vi "TANQUE_MAIN.vi"() -> ()   [LabVIEW 2017]
uses:
  <vilib>/Instr/_visa.llb/VISA Configure Serial Port (Instr).vi
  <vilib>/addons/database/Auxilliary.llb/DB Tools Format Datetime String (Time Stamp).vi
  <vilib>/addons/database/Connection.llb/DB Tools Open Connec (String).vi
  <vilib>/addons/database/NI_Database_API.lvlib
panel:
  out "SENSOR DE LLAMA":bool
  out "SENSOR DE PASO":bool
  out "hum":dbl
  out "tempp":dbl
  out "tanqueee":dbl
  in  "flow control":u16(ring) items=["None"=0, "XON/XOFF"=1, "RTS/CTS"=2, "DTR/DSR"=4]
  in  "stop bits":u16(ring)=10 items=["1.0"=10, "1.5"=15, "2.0"=20]
  in  "parity":u16(ring) items=["None", "Odd", "Even", "Mark", "Space"]
  in  "data bits":u16=8 min=5 max=8 step=1
  in  "VISA resource name":refnum<visa-resource-name>="COM1"
  in  "baud rate":u32=9600
  out "Humedity %":dbl(knob) scale=0.0..100.0
  out "Thermometer °C":dbl(slide) scale=0.0..50.0
  out "Tank":dbl(slide) scale=0.0..15.0
  out "DTH11":dbl(graph) caption="Canal Analogico 1"
  out "TERMOMETRO":dbl(graph) caption="Canal Analogico 1"
  out "ULTRASONIDO":dbl(graph) caption="Canal Analogico 1"
  # "Serial Port Config"
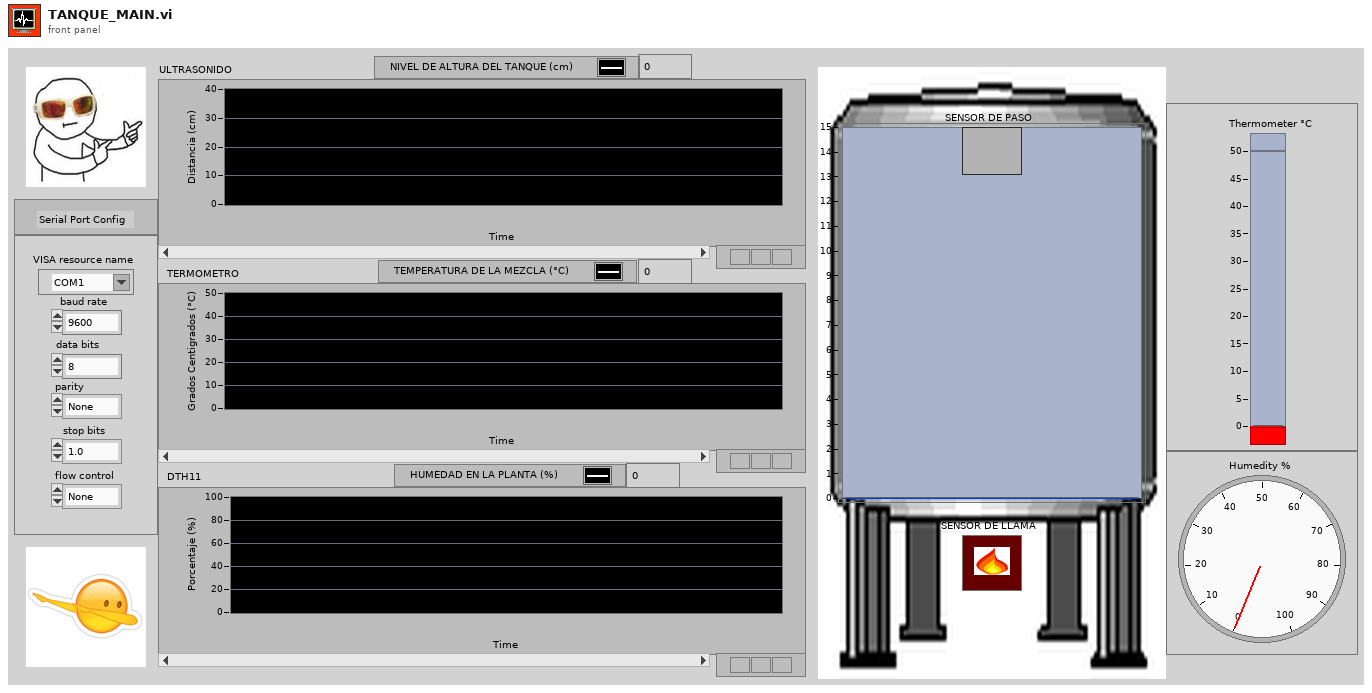
[diagram p1: front panel]
types:
  T1 = cluster{"unsigned byte array[0]":u8, "unsigned byte array[1]":u8, "unsigned byte array[2]":u8, "unsigned byte array[3]":u8, "unsigned byte array[4]":u8, "unsigned byte array[5]":u8}
  T2 = typedef "NI_Database_API.lvlib/Conn ObjectReference.ctl" = refnum<k1>
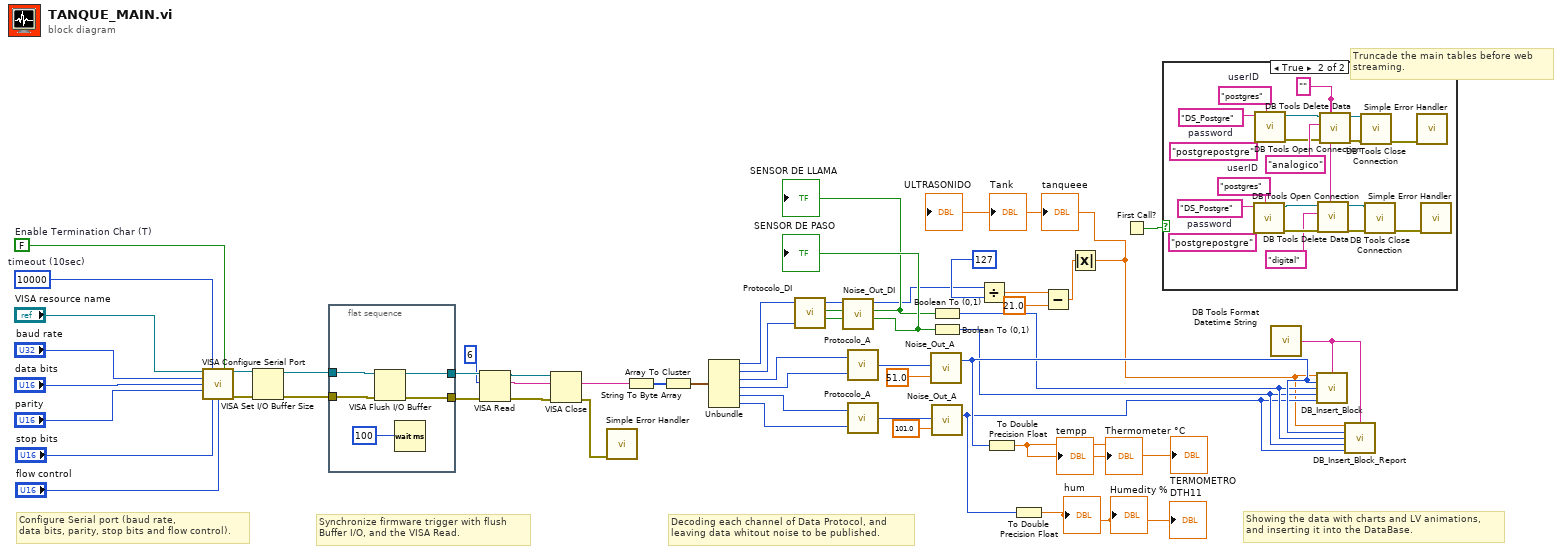
[diagram p0: block diagram]
diagram:
  w38 = FALSE  # Enable Termination Char (T)
  w39 = u32 10000  # timeout (10sec)
  # "Truncade the main tables before web \nstreaming."
  # "Showing the data with charts and LV animations,\nand inserting it into the DataBase."
  # "Decoding each channel of Data Protocol, and \nleaving data whitout noise to be published."
  # "Synchronize firmware trigger with flush \nBuffer I/O, and the VISA Read."
  # "Configure Serial port (baud rate,\ndata bits, parity, stop bits and flow control)."
  n1 = call-poly "VISA Configure Serial Port"("VISA resource name"="VISA resource name", "timeout (10sec)"=w39, "Enable Termination\nChar (T)"=w38, "baud rate (9600)"="baud rate", "data bits (8)"="data bits", "parity (0:none)"="parity", "stop bits (10: 1 bit)"="stop bits", "flow control (0:none)"="flow control") -> ("VISA resource name out"=w34:refnum<visa-resource-name>, "error out"=w33:errorcluster)  [unwired: 6 in]
  n2 = VISA Set I/O Buffer Size(VISA resource name=w34, error in (no error)=w33) -> (VISA resource name out=w32:refnum<visa-resource-name>, error out=w31:errorcluster)  [unwired: 2 in]
  n3 = flat-sequence {
    tunnel: w32 -> [w55]
    tunnel: w31 -> [w54]
    tunnel: [w53] -> w30
    tunnel: [w52] -> w29
    frame #0 {
      n4 = VISA Flush I/O Buffer(VISA resource name=w55, error in (no error)=w54) -> (VISA resource name out=w53:refnum<visa-resource-name>, error out=w52:errorcluster)  [unwired: 1 in]
      n5 = Wait (ms)(milliseconds to wait=u32 100) -> ()  [unwired: 1 out]
    }
  }
  n6 = VISA Read(VISA resource name=w30, byte count=u32 6, error in (no error)=w29) -> (VISA resource name out=w27:refnum<visa-resource-name>, read buffer=w25:string, error out=w26:errorcluster)  [unwired: 1 out]
  n7 = VISA Close(VISA resource name=w27, error in (no error)=w26) -> (error out=w28:errorcluster)
  n8 = call <vilib>:"Simple Error Handler.vi"("error in (no error)"=w28) -> ()  [unwired: 4 in, 5 out]
  n9 = String To Byte Array(string=w25) -> (unsigned byte array=w50:u8[])
  n10 = Array To Cluster(array=w50) -> (cluster=w49:T1)
  n11 = Unbundle(w49) -> ("unsigned byte array[0]"=w48:u8, "unsigned byte array[1]"=w47:u8, "unsigned byte array[2]"=w46:u8, "unsigned byte array[3]"=w45:u8, "unsigned byte array[4]"=w44:u8, "unsigned byte array[5]"=w43:u8)
  n12 = call "Protocolo_DI.vi"("Trama2"=w47, "Trama1"=w48) -> ("Digital2"=w9:bool, "Digital1"=w10:bool, "Analogico"=w11:u32)  [unwired: 1 in]
  n13 = call "Noise_Out_DI.vi"("D2"=w9, "D1"=w10, "IN"=w11) -> ("DOUT_2"=w14:bool, "DOUT_1"=w13:bool, "OUT"=w12:u32)  [unwired: 1 in, 1 out]
  "SENSOR DE PASO" <- w14
  "SENSOR DE LLAMA" <- w13
  n14 = call "Protocolo_A.vi"("Trama2"=w45, "Trama1"=w46) -> ("Analogico"=w18:u32)
  n15 = call "Protocolo_A.vi"("Trama2"=w43, "Trama1"=w44) -> ("Analogico"=w15:u32)
  n16 = call "Noise_Out_A.vi"("pico inalcanzable"=51.0, "IN"=w18) -> ("OUT"=w6:u32)  [unwired: 1 out]
  n17 = Boolean To (0,1)(Boolean=w13) -> (0, 1=w5:i16)
  n18 = Boolean To (0,1)(Boolean=w14) -> (0, 1=w4:i16)
  n19 = call "Noise_Out_A.vi"("pico inalcanzable"=101.0, "IN"=w15) -> ("OUT"=w3:u32)  [unwired: 1 out]
  n20 = Divide(x=w12, y=u32 127 ("x")) -> (x/y=w23:dbl)
  n21 = To Double Precision Float(number=w6) -> (double precision float=→"TERMOMETRO" →"Thermometer °C" →"tempp":dbl)
  n22 = To Double Precision Float(number=w3) -> (double precision float=→"DTH11" →"Humedity %" →"hum":dbl)
  n23 = Subtract(x=w23, y=21.0) -> (x-y=w2:dbl)
  n24 = Absolute Value(x=w2) -> (abs(x)=w1:dbl)
  "ULTRASONIDO" <- w1
  "Tank" <- w1
  "tanqueee" <- w1
  n25 = First Call?() -> (First Call?: T/F=w8:bool)
  n26 = case shown="True" w8 {
    frame False {
    }
    frame True {
      w56 = "" ("condition")
      (unwired) "postgrepostgre"  # password
      w70 = "postgres"  # userID
      (unwired) "postgrepostgre"  # password
      w72 = "postgres"  # userID
      n27 = call-poly <vilib>:"DB Tools Open Connection.vi"("userID"=w72, "connection information"="DS_Postgre") -> ("error out"=w65:errorcluster, "connection reference"=w64:T2)  [unwired: 6 in]
      n28 = call-poly <vilib>:"DB Tools Open Connection.vi"("userID"=w70, "connection information"="DS_Postgre") -> ("error out"=w66:errorcluster, "connection reference"=w67:T2)  [unwired: 6 in]
      n29 = call <vilib>:"DB Tools Delete Data.vi"("condition"=w56, "error in (no error)"=w65, "table"="digital", "connection reference"=w64) -> ("error out"=w59:errorcluster, "connection reference out"=w60:T2)  [unwired: 6 in]
      n30 = call <vilib>:"DB Tools Delete Data.vi"("condition"=w56, "error in (no error)"=w66, "table"="analogico", "connection reference"=w67) -> ("error out"=w58:errorcluster, "connection reference out"=w57:T2)  [unwired: 6 in]
      n31 = call <vilib>:"DB Tools Close Connection.vi"("error in (no error)"=w58, "connection reference"=w57) -> ("error out"=w62:errorcluster)  [unwired: 5 in]
      n32 = call <vilib>:"DB Tools Close Connection.vi"("error in (no error)"=w59, "connection reference"=w60) -> ("error out"=w61:errorcluster)  [unwired: 5 in]
      n33 = call <vilib>:"Simple Error Handler.vi"("error in (no error)"=w62) -> ()  [unwired: 4 in, 5 out]
      n34 = call <vilib>:"Simple Error Handler.vi"("error in (no error)"=w61) -> ()  [unwired: 4 in, 5 out]
    }
  }
  n35 = call-poly <vilib>:"DB Tools Format Datetime String.vi"() -> ("date/time string"=w7:string)  [unwired: 1 in]
  n36 = call "DB_Insert_Block.vi"("Numeric (DATO)"=w1, "date/time string"=w7, "Numeric (DATO) 2"=w6, "BIT (DATO)"=w5, "BIT (DATO) 2"=w4, "Numeric (DATO) 3"=w3) -> ()  [unwired: 10 in]
  n37 = call "DB_Insert_Block_Report.vi"("Numeric (DATO)"=w1, "date/time string"=w7, "Numeric (DATO) 2"=w6, "BIT (DATO)"=w5, "BIT (DATO) 2"=w4, "Numeric (DATO) 3"=w3) -> ()  [unwired: 10 in]
